vi "Query Parameter XML File - 1553.vi"(0 "Path in":path=path "C:/work/SE/Opportunities/2012/Pilatus/201210/TestXMLs/Receiver.xml", 5 "Bus Without Parms":T1, 11 "error in (no error)":errorcluster) -> (6 "Bus With Parms":T1, 15 "error out":errorcluster)   [LabVIEW 2013, in "AIT 1553 Custom Device.lvlib"]
uses:
  AIT 1553 Custom Device.lvlib
  Controls/1553_Bus.ctl
  Controls/1553_Bus_Controller.ctl
  Controls/1553_BC_Message.ctl
  Controls/1553 Param.ctl
  Controls/1553_Acyclic_Frame.ctl
  Controls/1553_Bus_Monitor.ctl
  Controls/1553_BM_Message.ctl
  Controls/1553_RT_Message.ctl
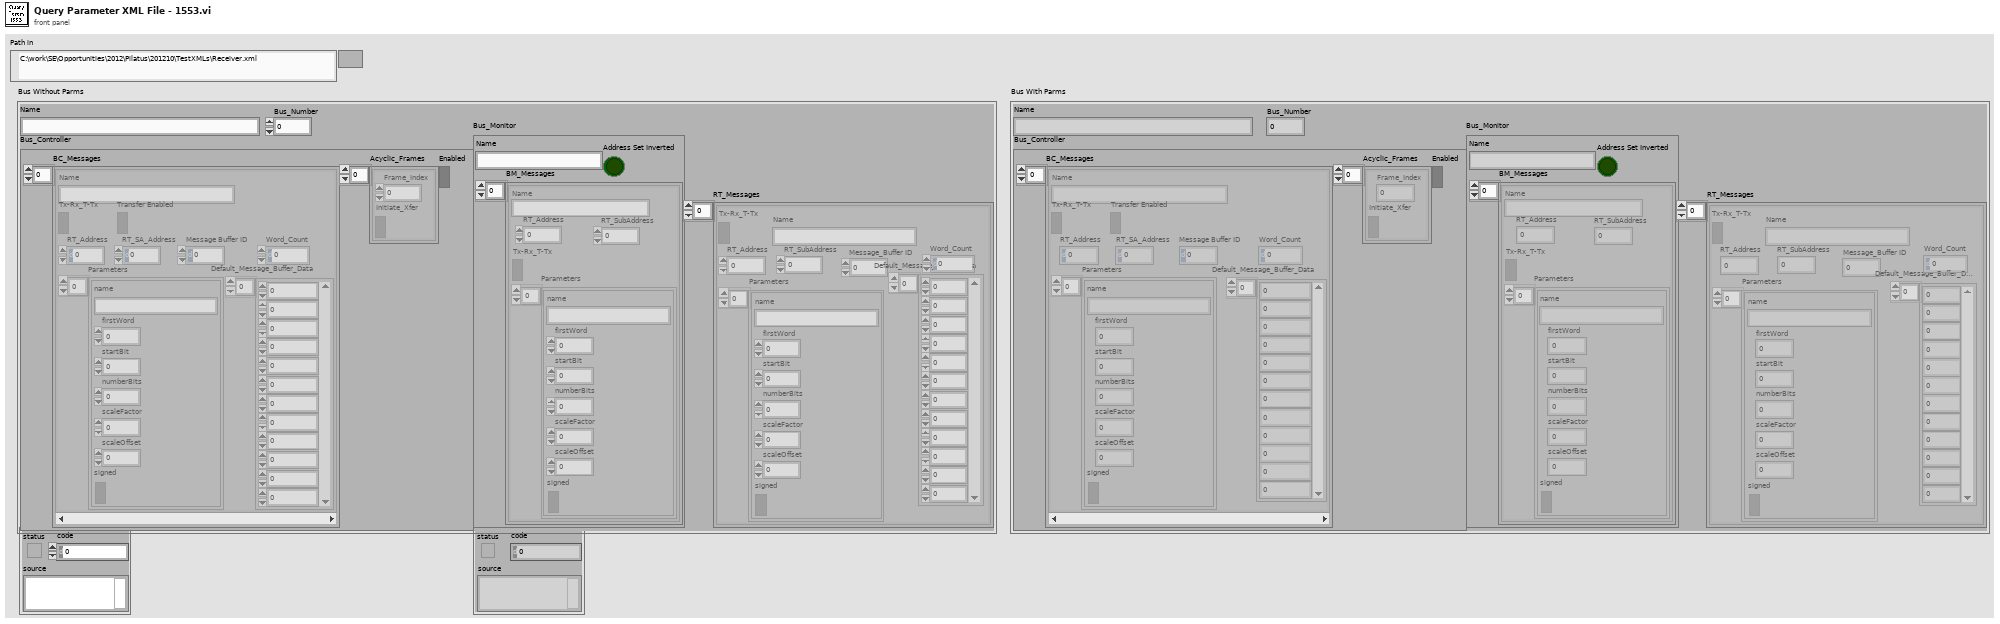
[diagram p1: front panel]
types:
  T1 = typedef "AIT 1553 Custom Device.lvlib/1553_Bus.ctl" = cluster{"Name":string, "Bus_Number":u8, "Bus_Controller":T2, "Bus_Monitor":T6, "RT_Messages":T8[]}
  T2 = typedef "AIT 1553 Custom Device.lvlib/1553_Bus_Controller.ctl" = cluster{"BC_Messages":T3[], "Acyclic_Frames":T5[], "Enabled":bool}
  T3 = typedef "AIT 1553 Custom Device.lvlib/1553_BC_Message.ctl" = cluster{"Name":string, "Tx-Rx_T-Tx":bool, "RT_Address":u8, "RT_SA_Address":u8, "Parameters":T4[], "Transfer Enabled":bool, "Message Buffer ID":u16, "Default_Message_Buffer_Data":u16[], "Word_Count":u8}
  T4 = typedef "AIT 1553 Custom Device.lvlib/1553 Param.ctl" = cluster{"name":string, "firstWord":i32, "startBit":i32, "numberBits":i32, "scaleFactor":dbl, "scaleOffset":dbl, "signed":bool}
  T5 = typedef "AIT 1553 Custom Device.lvlib/1553_Acyclic_Frame.ctl" = cluster{"Frame_Index":u8, "Initiate_Xfer":bool}
  T6 = typedef "AIT 1553 Custom Device.lvlib/1553_Bus_Monitor.ctl" = cluster{"Name":string, "BM_Messages":T7[], "Address Set Inverted":bool}
  T7 = typedef "AIT 1553 Custom Device.lvlib/1553_BM_Message.ctl" = cluster{"RT_Address":u8, "RT_SubAddress":u8, "Tx-Rx_T-Tx":bool, "Parameters":T4[], "Name":string}
  T8 = typedef "AIT 1553 Custom Device.lvlib/1553_RT_Message.ctl" = cluster{"RT_Address":u8, "RT_SubAddress":u8, "Tx-Rx_T-Tx":bool, "Parameters":T4[], "Message_Buffer ID":u16, "Default_Message_Buffer_Data":u16[], "Word_Count":u8, "Name":string}
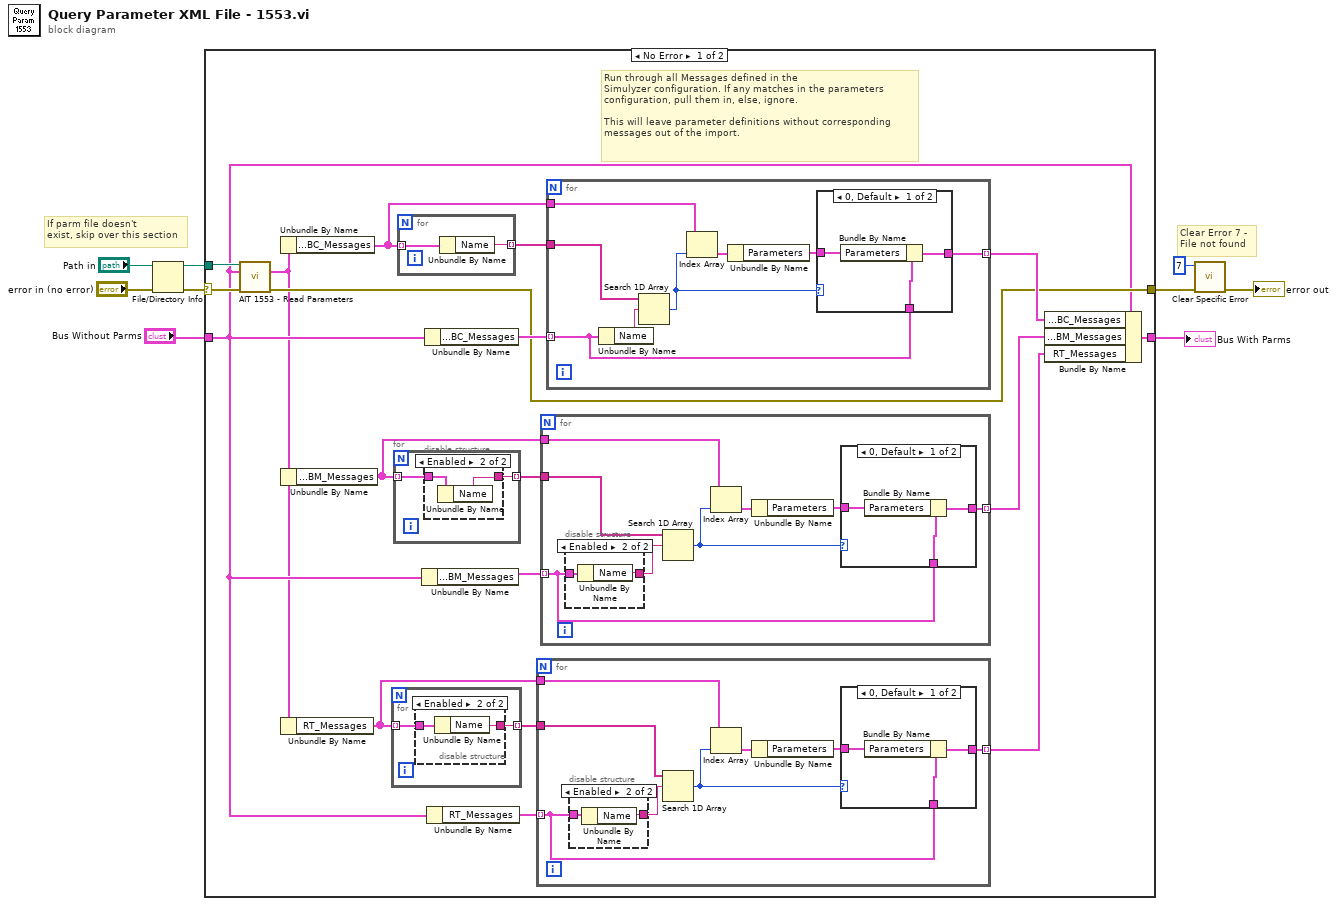
[diagram p0: block diagram]
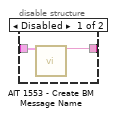
[diagram p2: hidden frame]
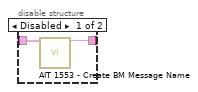
[diagram p4: hidden frame]
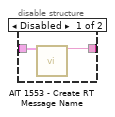
[diagram p5: hidden frame]
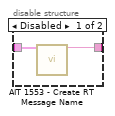
[diagram p8: hidden frame]
diagram:
  # "If parm file doesn't\nexist, skip over this section"
  # "Clear Error 7 - \nFile not found"
  n1 = File/Directory Info(path="Path in", error in="error in (no error)") -> (path out=w8:path, error out=w4:errorcluster)  [unwired: 5 out]
  n2 = case shown="No Error" w4 {
    selector: w4 -> [w22 w86]
    tunnel: [w18 w87] -> w9
    tunnel: w8 -> [w23 _]
    tunnel: [w17 w86] -> w6
    tunnel: "Bus Without Parms" -> [w16 w87]
    frame No Error {
      # "Run through all Messages defined in the\nSimulyzer configuration. If any matches in the parameters\nconfiguration, pull them in, else, ignore.\n\nThis will leave parameter definitions without corresponding\nmessages out of the import."
      n3 = call "AIT 1553 - Read Parameters.vi"("File Path"=w23, "Bus In"=w16, "error in (no error)"=w22) -> ("Bus Out"=w10:T1, "error out"=w17:errorcluster)  [unwired: 11 in]
      n4 = Unbundle By Name(w10) -> ("Bus_Controller.BC_Messages"=w26:T3[])
      n5 = Unbundle By Name(w10) -> ("Bus_Monitor.BM_Messages"=w14:T7[])
      n6 = Unbundle By Name(w10) -> ("RT_Messages"=w25:T8[])
      n7 = for {
        tunnel: w25 -> [w79] mode=indexing
        tunnel: [w78] -> w24 mode=indexing
        n8 = disable-structure shown="Enabled" {
          disable-tunnel: w79 -> [w81 w83]
          disable-tunnel: [w80 w82] -> w78
          frame Disabled {
            n9 = call "AIT 1553 - Create RT Message Name.vi"("RT_Message"=w81) -> ("Message Name"=w80:string)  [unwired: 13 in, 1 out]
          }
          frame Enabled {
            n10 = Unbundle By Name(w83) -> ("Name"=w82:string)
          }
        }
      }
      n11 = for {
        tunnel: w14 -> [w45] mode=indexing
        tunnel: [w44] -> w12 mode=indexing
        n12 = disable-structure shown="Enabled" {
          disable-tunnel: w45 -> [w47 w49]
          disable-tunnel: [w46 w48] -> w44
          frame Disabled {
            n13 = call "AIT 1553 - Create BM Message Name.vi"("BM_Message"=w47) -> ("Message Name"=w46:string)  [unwired: 13 in, 1 out]
          }
          frame Enabled {
            n14 = Unbundle By Name(w49) -> ("Name"=w48:string)
          }
        }
      }
      n15 = for {
        tunnel: w26 -> [w85] mode=indexing
        tunnel: [w84] -> w27 mode=indexing
        n16 = Unbundle By Name(w85) -> ("Name"=w84:string)
      }
      n17 = Unbundle By Name(w16) -> ("Bus_Monitor.BM_Messages"=w13:T7[])
      n18 = Unbundle By Name(w16) -> ("Bus_Controller.BC_Messages"=w21:T3[])
      n19 = Unbundle By Name(w16) -> ("RT_Messages"=w20:T8[])
      n20 = for {
        tunnel: w20 -> [w52] mode=indexing
        tunnel: w24 -> [w50]
        tunnel: [w57] -> w15 mode=indexing
        tunnel: w25 -> [w56]
        n21 = disable-structure shown="Enabled" {
          disable-tunnel: w52 -> [w59 w61]
          disable-tunnel: [w58 w60] -> w51
          frame Disabled {
            n22 = call "AIT 1553 - Create RT Message Name.vi"("RT_Message"=w59) -> ("Message Name"=w58:string)  [unwired: 13 in, 1 out]
          }
          frame Enabled {
            n23 = Unbundle By Name(w61) -> ("Name"=w60:string)
          }
        }
        n24 = Search 1D Array(1D array=w50, element=w51) -> (index of element=w55:i32)  [unwired: 1 in]
        n25 = Index Array(array=w56, index=w55) -> (element=w54:T8)
        n26 = Unbundle By Name(w54) -> ("Parameters"=w53:T4[])
        n27 = case shown="0, Default" w55 {
          tunnel: w53 -> [w64 _]
          tunnel: [w63 w65] -> w57
          tunnel: w52 -> [w62 w65]
          frame 0, Default {
            n28 = Bundle By Name(cluster=w62, "Parameters"=w64) -> (w63:T8)
          }
          frame -1 {
          }
        }
      }
      n29 = for {
        tunnel: w13 -> [w29] mode=indexing
        tunnel: w12 -> [w33]
        tunnel: [w35] -> w11 mode=indexing
        tunnel: w14 -> [w34]
        n30 = disable-structure shown="Enabled" {
          disable-tunnel: w29 -> [w37 w39]
          disable-tunnel: [w36 w38] -> w28
          frame Disabled {
            n31 = call "AIT 1553 - Create BM Message Name.vi"("BM_Message"=w37) -> ("Message Name"=w36:string)  [unwired: 13 in, 1 out]
          }
          frame Enabled {
            n32 = Unbundle By Name(w39) -> ("Name"=w38:string)
          }
        }
        n33 = Search 1D Array(1D array=w33, element=w28) -> (index of element=w32:i32)  [unwired: 1 in]
        n34 = Index Array(array=w34, index=w32) -> (element=w31:T7)
        n35 = Unbundle By Name(w31) -> ("Parameters"=w30:T4[])
        n36 = case shown="0, Default" w32 {
          tunnel: w30 -> [w42 _]
          tunnel: [w41 w43] -> w35
          tunnel: w29 -> [w40 w43]
          frame 0, Default {
            n37 = Bundle By Name(cluster=w40, "Parameters"=w42) -> (w41:T7)
          }
          frame -1 {
          }
        }
      }
      n38 = for {
        tunnel: w21 -> [w71] mode=indexing
        tunnel: w27 -> [w69]
        tunnel: [w73] -> w19 mode=indexing
        tunnel: w26 -> [w70]
        n39 = Unbundle By Name(w71) -> ("Name"=w72:string)
        n40 = Search 1D Array(1D array=w69, element=w72) -> (index of element=w68:i32)  [unwired: 1 in]
        n41 = Index Array(array=w70, index=w68) -> (element=w67:T3)
        n42 = Unbundle By Name(w67) -> ("Parameters"=w66:T4[])
        n43 = case shown="0, Default" w68 {
          tunnel: w66 -> [w76 _]
          tunnel: [w75 w77] -> w73
          tunnel: w71 -> [w74 w77]
          frame 0, Default {
            n44 = Bundle By Name(cluster=w74, "Parameters"=w76) -> (w75:T3)
          }
          frame -1 {
          }
        }
      }
      n45 = Bundle By Name(cluster=w16, "Bus_Controller.BC_Messages"=w19, "Bus_Monitor.BM_Messages"=w11, "RT_Messages"=w15) -> (w18:T1)
    }
    frame Error {
    }
  }
  "Bus With Parms" <- w9
  n46 = call "Clear Specific Error.vi"("error in (no error)"=w6, "code"=7) -> ("error out"=→"error out":errorcluster)  [unwired: 8 in, 1 out]
